vi "niRFUtil WFM Pad Waveform (complex wfm).vi"(0 "Waveform In":T2 {"y" format="%.2f"; "dx" format="%^.2e"; "x0" format="%^.2e"}, 2 "Padding Type (Zero)":T1(ring), 13 "Duration":dbl format="%^.2e") -> (4 "Waveform Out":T2 {"y" format="%.2f"; "dx" format="%^.2e"; "x0" format="%^.2e"})   [LabVIEW 2015, in "niRFUtil.lvlib"]
doc: "(c) Copyright 2006, National Instruments, Inc. This VI may not be duplicated, sold, or distributed without written consent from National Instruments."
uses:
  niRFUtil.lvlib
  Includes/niRFUtil INC Complex Waveform.ctl
  Includes/niRFUtil INC Complex Array.ctl
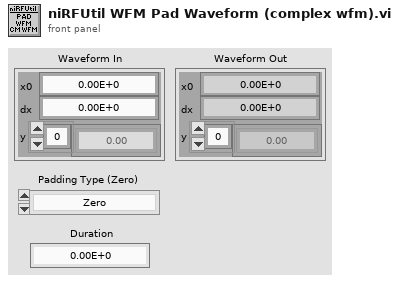
[diagram p1: front panel]
types:
  T1 = enum16{"Zero", "Leading/Trailing", "Cyclic Prefix/Postfix"}
  T2 = typedef "niRFUtil.lvlib/niRFUtil INC Complex Waveform.ctl" = cluster{"x0":dbl, "dx":dbl, "y":T3}
  T3 = typedef "niRFUtil.lvlib/niRFUtil INC Complex Array.ctl" = csg[]
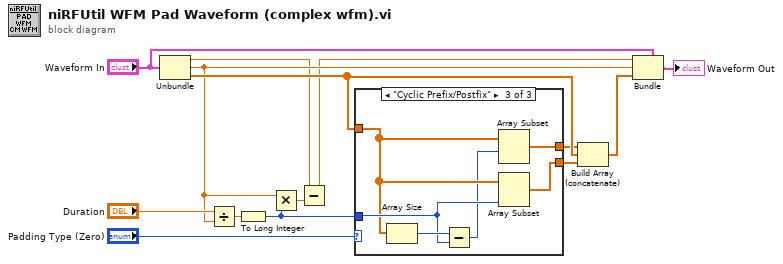
[diagram p0: block diagram]
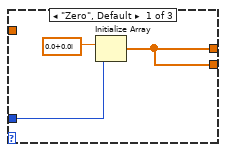
[diagram p2: hidden frame]
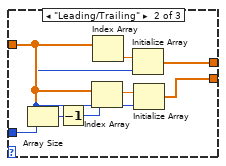
[diagram p3: hidden frame]
diagram:
  n1 = Unbundle("Waveform In") -> ("x0"=w3:dbl, "dx"=w5:dbl, "y"=w11:T3)
  n2 = Divide(x="Duration", y=w5) -> (x/y=w14:dbl)
  n3 = To Long Integer(number=w14) -> (32bit integer=w6:i32)
  n4 = Multiply(x=w5, y=w6) -> (x*y=w4:dbl)
  n5 = Subtract(x=w3, y=w4) -> (x-y=w2:dbl)
  n6 = case shown="\"Cyclic Prefix/Postfix\"" "Padding Type (Zero)" {
    tunnel: w6 -> [w16 w18 w30]
    tunnel: [w17 w19 w26] -> w12
    tunnel: w11 -> [_ w20 w29]
    tunnel: [w17 w24 w27] -> w10
    frame "Zero", Default {
      n7 = Initialize Array(csg 0.0+0.0i ("Numeric"), w16) -> (w17:csg[])
    }
    frame "Leading/Trailing" {
      n8 = Array Size(array=w20) -> (size(s)=w22:i32)
      n9 = Decrement(x=w22) -> (x-1=w21:i32)
      n10 = Index Array(array=w20, index=w21) -> (element=w23:csg)
      n11 = Index Array(array=w20) -> (element=w25:csg)  [unwired: 1 in]
      n12 = Initialize Array(w25, w18) -> (w24:csg[])
      n13 = Initialize Array(w23, w18) -> (w19:csg[])
    }
    frame "Cyclic Prefix/Postfix" {
      n14 = Array Size(array=w29) -> (size(s)=w31:i32)
      n15 = Subtract(x=w31, y=w30) -> (x-y=w28:i32)
      n16 = Array Subset(array=w29, index=w28) -> (w27:T3)  [unwired: 1 in]
      n17 = Array Subset(array=w29, length=w30) -> (w26:T3)  [unwired: 1 in]
    }
  }
  n18 = Build Array (concatenate)(w10, w11, w12) -> (w13:T3)
  n19 = Bundle(cluster="Waveform In", "x0"=w2, "dx"=w5, "y"=w13) -> (→"Waveform Out":T2)
